vi "RichToFlatnixnet_grpc_ReadFrameResponse.vi"(5 "OutputClusterType":T1, 11 "InputCluster":T9) -> (3 "OutputCluster":T1)   [LabVIEW 2025, in "grpc-xnet_client.lvlib"]
uses:
  nixnet_grpc_ReadFrameResponse.ctl
  nixnet_grpc_FrameBufferResponse.ctl
  nixnet_grpc_FrameBufferResponse_frame/nixnet_grpc_FrameBufferResponse_frame.lvclass
  nixnet_grpc_ReadFrameResponse_Flat.ctl
  nixnet_grpc_FrameBufferResponse_Flat.ctl
  nixnet_grpc_FrameResponse_Flat.ctl
  nixnet_grpc_FrameType.ctl
  nixnet_grpc_FrameFlags.ctl
  nixnet_grpc_EnetFrameResponse_Flat.ctl
  nixnet_grpc_EnetFrameType.ctl
  nixnet_grpc_EnetFlags.ctl
  grpc-xnet_client.lvlib
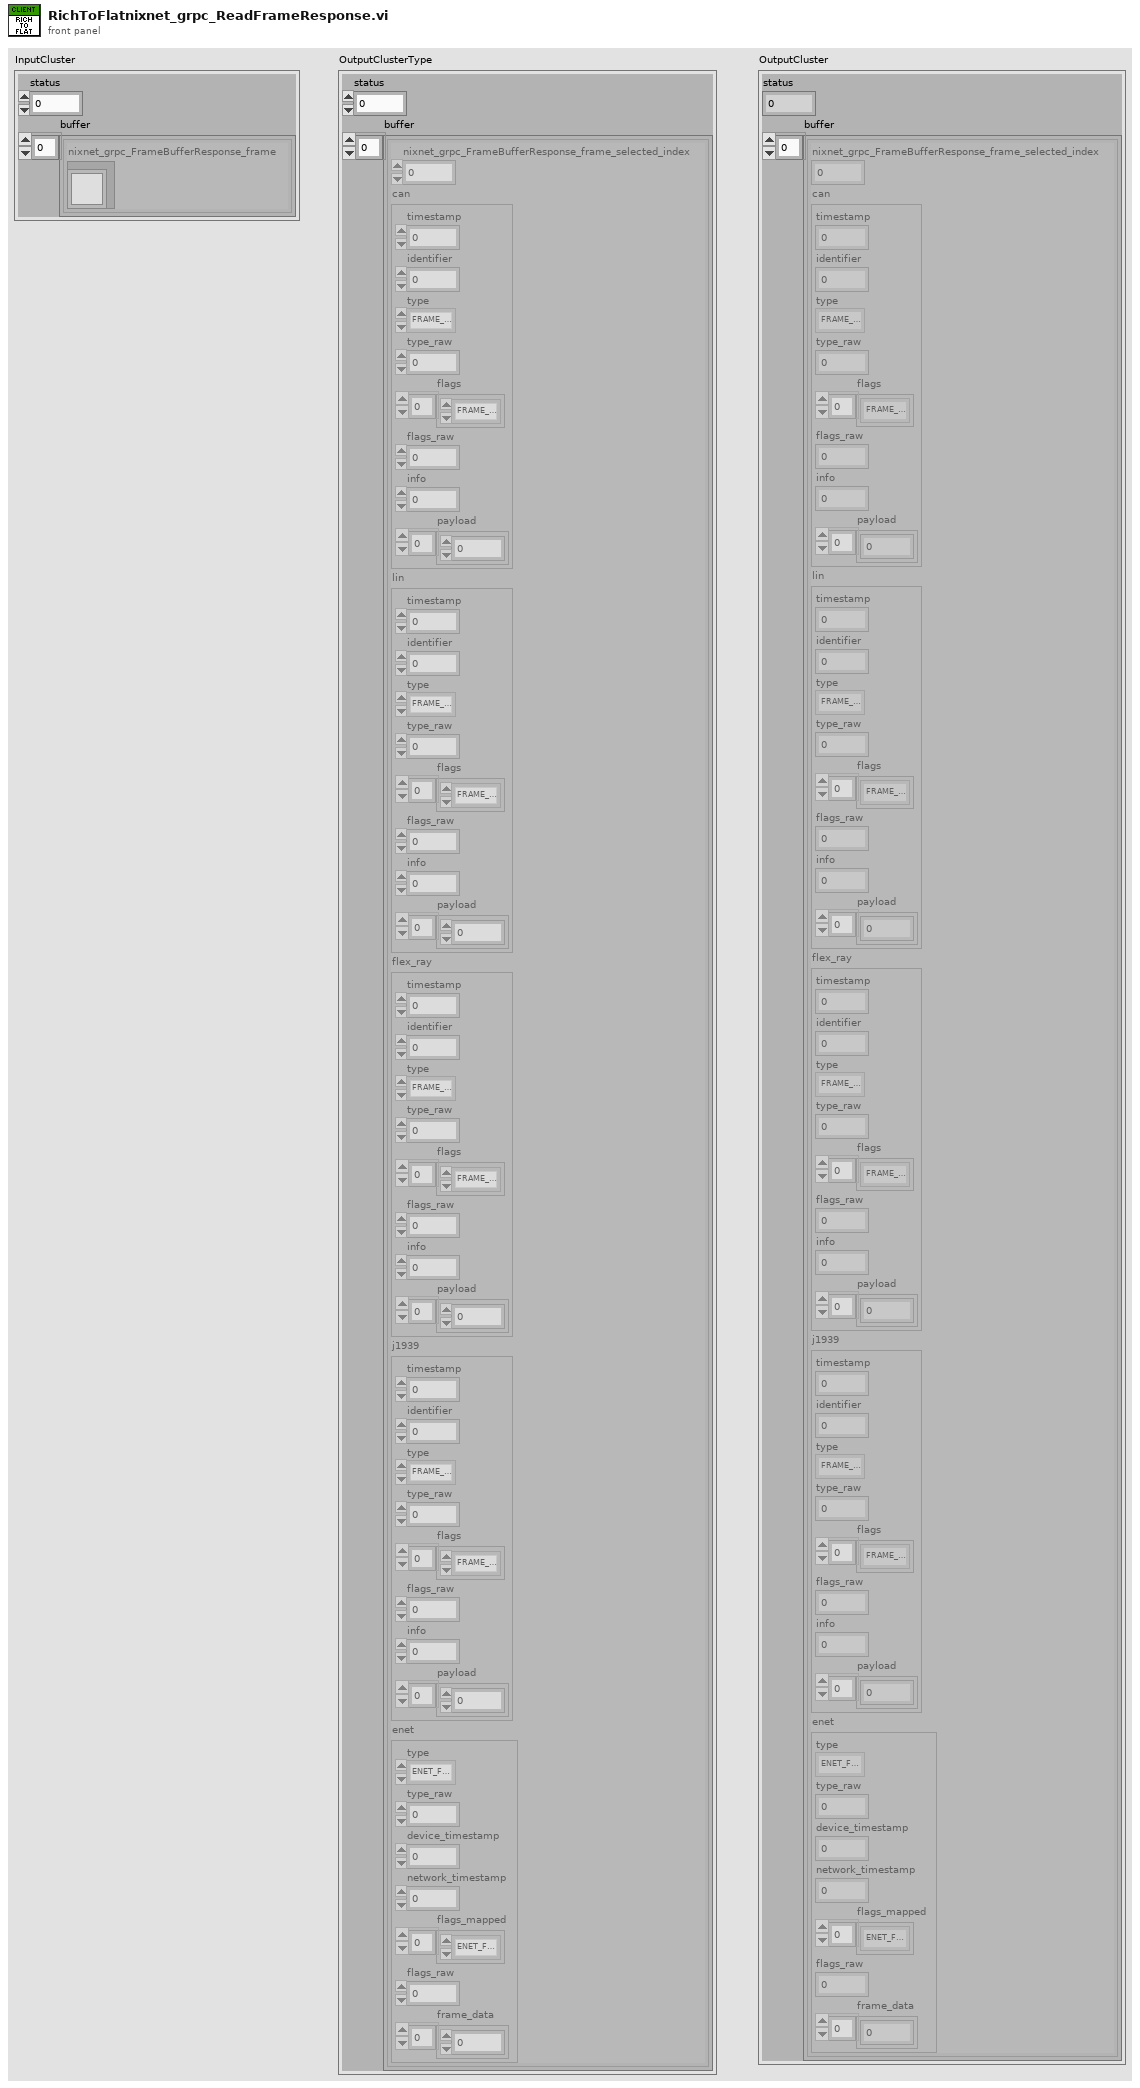
[diagram p1: front panel]
types:
  T1 = typedef "grpc-xnet_client.lvlib/nixnet_grpc_ReadFrameResponse_Flat.ctl" = cluster{"status":i32, "buffer":T2[]}
  T2 = typedef "grpc-xnet_client.lvlib/nixnet_grpc_FrameBufferResponse_Flat.ctl" = cluster{"nixnet_grpc_FrameBufferResponse_frame_selected_index":i32, "can":T3, "lin":T3, "flex_ray":T3, "j1939":T3, "enet":T6}
  T3 = typedef "grpc-xnet_client.lvlib/nixnet_grpc_FrameResponse_Flat.ctl" = cluster{"timestamp":u64, "identifier":u32, "type":T4, "type_raw":u32, "flags":T5[], "flags_raw":u32, "info":u32, "payload":u8[]}
  T4 = typedef "grpc-xnet_client.lvlib/nixnet_grpc_FrameType.ctl" = enum32{"FRAME_TYPE_CAN_DATA", "FRAME_TYPE_CAN_REMOTE", "FRAME_TYPE_CAN_BUS_ERROR", "FRAME_TYPE_CAN20_DATA", "FRAME_TYPE_CANFD_DATA", "FRAME_TYPE_CANFDBRS_DATA", "FRAME_TYPE_FLEX_RAY_DATA", "FRAME_TYPE_FLEX_RAY_NULL", "FRAME_TYPE_FLEX_RAY_SYMBOL", "FRAME_TYPE_LIN_DATA", "FRAME_TYPE_LIN_BUS_ERROR", "FRAME_TYPE_LIN_NO_RESPONSE", "FRAME_TYPE_J1939_DATA", "FRAME_TYPE_SPECIAL_DELAY", "FRAME_TYPE_SPECIAL_LOG_TRIGGER", "FRAME_TYPE_SPECIAL_START_TRIGGER"}
  T5 = typedef "grpc-xnet_client.lvlib/nixnet_grpc_FrameFlags.ctl" = enum32{"FRAME_FLAGS_UNSPECIFIED", "FRAME_FLAGS_FLEX_RAY_STARTUP", "FRAME_FLAGS_FLEX_RAY_SYNC", "FRAME_FLAGS_FLEX_RAY_PREAMBLE", "FRAME_FLAGS_FLEX_RAY_CH_A", "FRAME_FLAGS_FLEX_RAY_CH_B", "FRAME_FLAGS_LIN_EVENT_SLOT", "FRAME_FLAGS_TRANSMIT_ECHO"}
  T6 = typedef "grpc-xnet_client.lvlib/nixnet_grpc_EnetFrameResponse_Flat.ctl" = cluster{"type":T7, "type_raw":u32, "device_timestamp":u64, "network_timestamp":u64, "flags_mapped":T8[], "flags_raw":u32, "frame_data":u8[]}
  T7 = typedef "grpc-xnet_client.lvlib/nixnet_grpc_EnetFrameType.ctl" = enum32{"ENET_FRAME_TYPE_DATA", "ENET_FRAME_TYPE_DELAY", "ENET_FRAME_TYPE_FUTURE_TIME_WAIT"}
  T8 = typedef "grpc-xnet_client.lvlib/nixnet_grpc_EnetFlags.ctl" = enum32{"ENET_FLAGS_UNSPECIFIED", "ENET_FLAGS_TRANSMIT", "ENET_FLAGS_RECEIVE", "ENET_FLAGS_NETWORK_SYNCED", "ENET_FLAGS_ERROR"}
  T9 = typedef "grpc-xnet_client.lvlib/nixnet_grpc_ReadFrameResponse.ctl" = cluster{"status":i32, "buffer":T10[]}
  T10 = typedef "grpc-xnet_client.lvlib/nixnet_grpc_FrameBufferResponse.ctl" = cluster{"nixnet_grpc_FrameBufferResponse_frame":refnum<class "nixnet_grpc_FrameBufferResponse_frame.lvclass">}
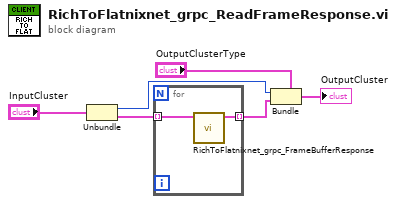
[diagram p0: block diagram]
diagram:
  n1 = Unbundle "Unbundle"("InputCluster") -> ("status"=w3:i32, "buffer"=w2:T10[])
  n2 = for {
    tunnel: w2 -> [w8] mode=indexing
    tunnel: [w7] -> w1 mode=indexing
    n3 = call "RichToFlatnixnet_grpc_FrameBufferResponse.vi"("InputCluster"=w8) -> ("OutputCluster"=w7:T2)  [unwired: 10 in]
  }
  n4 = Bundle "Bundle"(cluster="OutputClusterType", "status"=w3, "buffer"=w1) -> (→"OutputCluster":T1)
